vi "Inst.Magneto.GetPrivateEvents.vi"(8 "error in (no error)":errorcluster, 11 "Inst.Magneto in":refnum<class "Inst.Magneto.lvclass">) -> (0 "error out":errorcluster, 2 "Inst.Magneto Private Events":cluster{"MessageToProcess":refnum<user-event>}, 3 "Inst.Magneto out":refnum<class "Inst.Magneto.lvclass">)   [LabVIEW 2019, in "Inst.Magneto.lvclass"]
uses:
  Inst.Magneto.lvclass
  Typedefs/PrivateEvents--Inst.Magneto.MessageToProcess.ctl
  <userlib>/Levylab/Instrument Framework/SMOs/RemoteControl/Typedefs/Message--Cluster.ctl
  Inst.Magneto.lvclass/Inst.Magneto.ctl
  <userlib>/Levylab/Instrument Framework/SMOs/RemoteControl/RemoteControl.lvclass
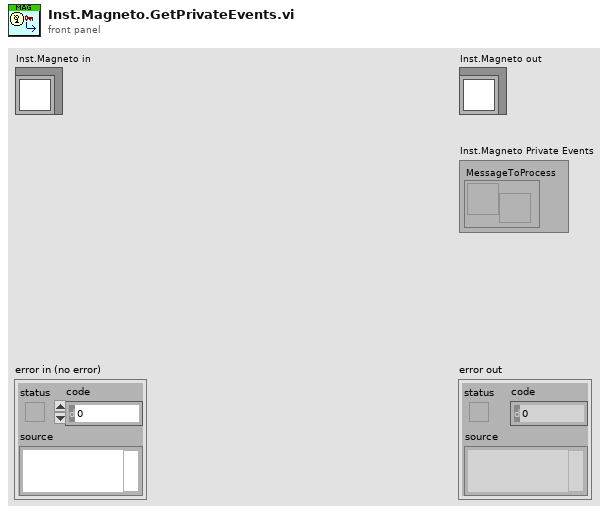
[diagram p1: front panel]
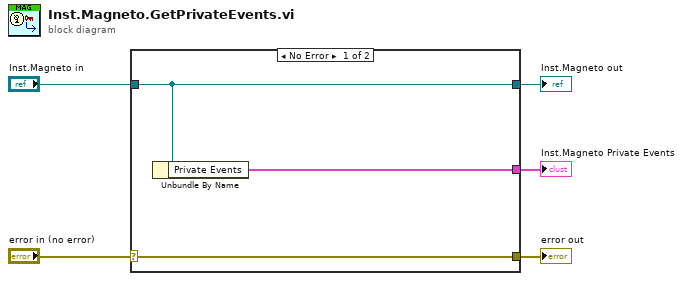
[diagram p0: block diagram]
diagram:
  n1 = case shown="No Error" "error in (no error)" {
    selector: "error in (no error)" -> [w8 w9]
    tunnel: [w8 w9] -> w4
    tunnel: [w7 w10] -> w2
    tunnel: "Inst.Magneto in" -> [w7 w10]
    tunnel: [w6 _] -> w1
    frame No Error {
      n2 = Unbundle By Name(w7) -> ("Private Events"=w6:cluster{"MessageToProcess":refnum<user-event>})
    }
    frame Error {
    }
  }
  "error out" <- w4
  "Inst.Magneto out" <- w2
  "Inst.Magneto Private Events" <- w1
